vi "LogQueue.vi"() -> (3 "LogQueue":T1)   [LabVIEW 2018]
uses:
  LogDataQueue.ctl
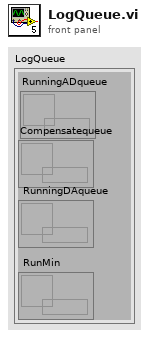
[diagram p1: front panel]
types:
  T1 = typedef "LogDataQueue.ctl" = cluster{"RunningADqueue":refnum<queue>, "Compensatequeue":refnum<queue>, " RunningDAqueue":refnum<queue>, " RunMin":refnum<queue>}
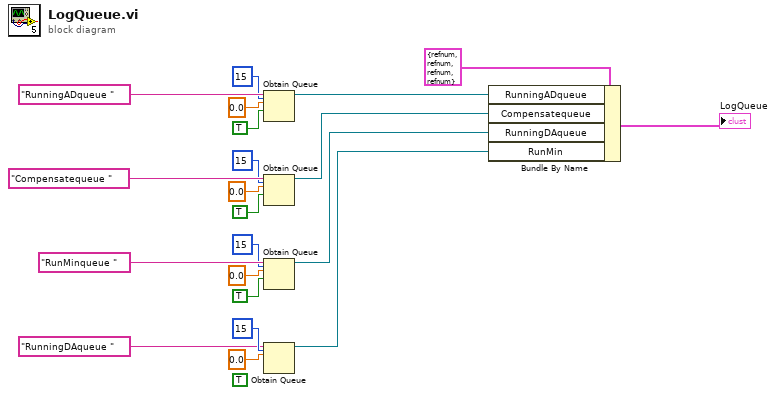
[diagram p0: block diagram]
diagram:
  (unwired) TRUE ("如未找到则创建？(T)")
  n1 = Obtain Queue(max queue size (-1, unlimited)=15 ("中值标准差队列长度"), name (unnamed)="RunningADqueue " ("名称（未命名）"), element data type=0.0, create if not found? (T)=TRUE ("如未找到则创建？(T)")) -> (queue out=w12:refnum<queue>)  [unwired: 1 in, 2 out]
  n2 = Obtain Queue(max queue size (-1, unlimited)=15 ("中值标准差队列长度"), name (unnamed)="Compensatequeue " ("名称（未命名）"), element data type=0.0, create if not found? (T)=TRUE ("如未找到则创建？(T)")) -> (queue out=w13:refnum<queue>)  [unwired: 1 in, 2 out]
  n3 = Obtain Queue(max queue size (-1, unlimited)=15 ("中值标准差队列长度"), name (unnamed)="RunMinqueue " ("名称（未命名）"), element data type=0.0, create if not found? (T)=TRUE ("如未找到则创建？(T)")) -> (queue out=w14:refnum<queue>)  [unwired: 1 in, 2 out]
  n4 = Obtain Queue(max queue size (-1, unlimited)=15 ("中值标准差队列长度"), name (unnamed)="RunningDAqueue " ("名称（未命名）"), element data type=0.0) -> (queue out=w15:refnum<queue>)  [unwired: 2 in, 2 out]
  n5 = Bundle By Name(cluster=T1 {"RunningADqueue"=refnum, "Compensatequeue"=refnum, " RunningDAqueue"=refnum, " RunMin"=refnum} ("输入簇"), "RunningADqueue"=w12, "Compensatequeue"=w13, "RunningDAqueue"=w14, "RunMin"=w15) -> (→"LogQueue":T1)
